vi "macro_DrumSeq_Pulse_Mux.vi"   [LabVIEW 2019, in "Trajectory_Library.lvlib"]
uses:
  VI/BoolCmd_Recv_Internal.vi
  VI/DigSeqLogic_Edge_On.vi
  VI/BoolCmd_ObtainQueue.vi
  Trajectory_Library.lvlib
types:
  T1 = typedef "Trajectory_Library.lvlib/DrumSequence_Step_Enum.ctl" = enum16{"Do Nothing", "Step 1", "Step 2", "Step 3", "Step 4", "Step 5", "Step 6", "Step 7", "Step 8", "Step 9", "Step 10", "Step 11", "Step 12", "Step 13", "Step 14", "Step 15", "Step 16", "Step 17", "Step 18", "Step 19", "Step 20", "Step 21", "Step 22", "Step 23", "Step 24", "Step 25", "Step 26", "Step 27", "Step 28", "Step 29", "Step 30", "Step 31", "Step 32", "Cancel", "Initialize", "Error"}
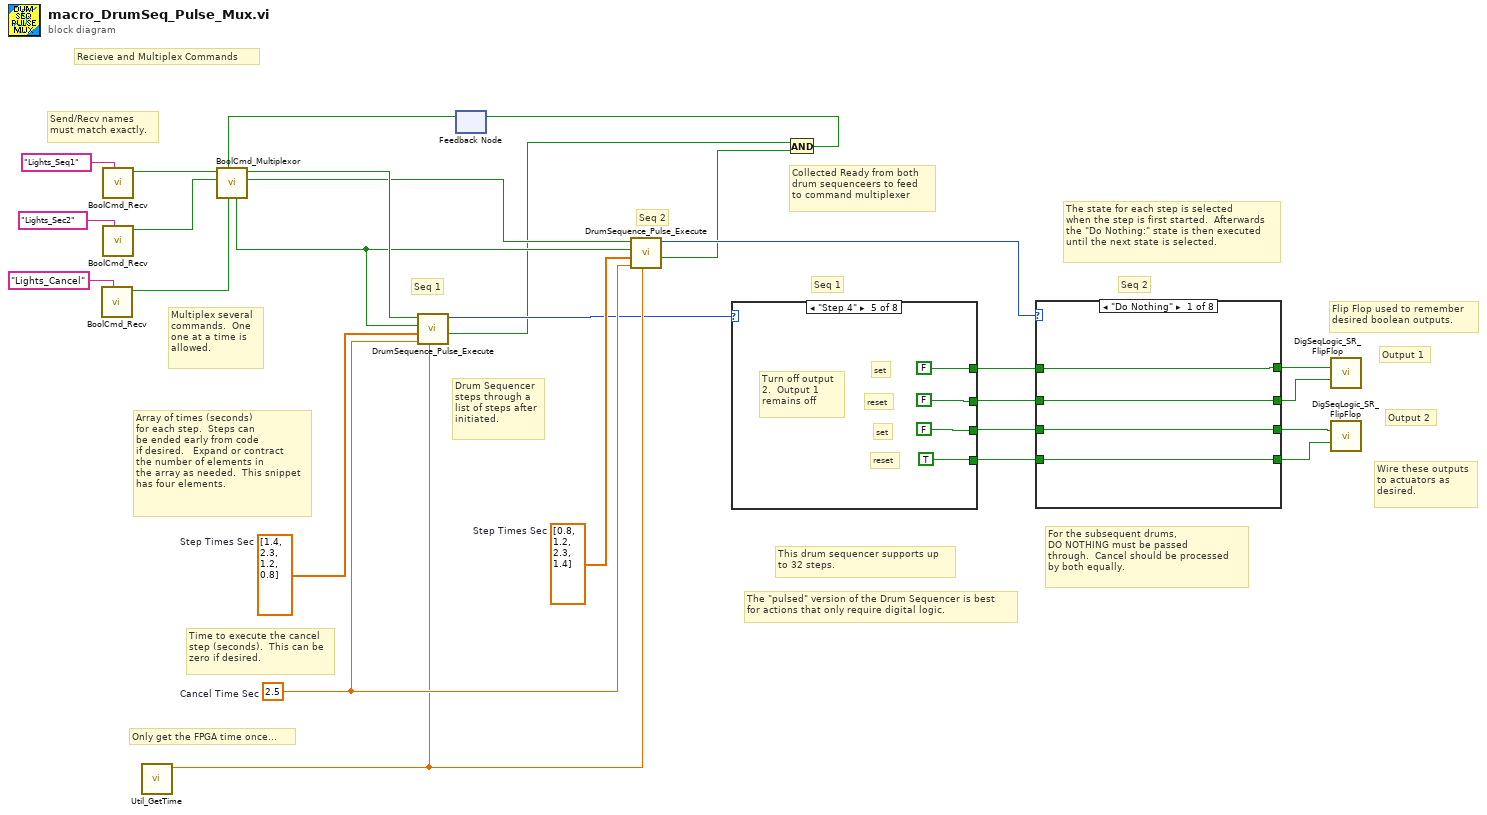
[diagram p0: block diagram]
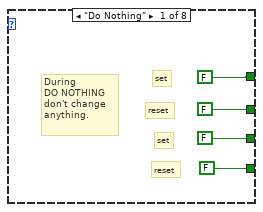
[diagram p2: hidden frame]
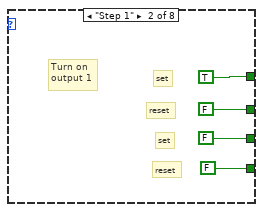
[diagram p3: hidden frame]
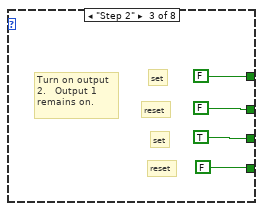
[diagram p4: hidden frame]
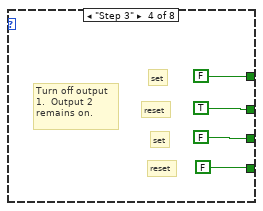
[diagram p5: hidden frame]
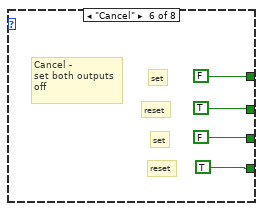
[diagram p6: hidden frame]
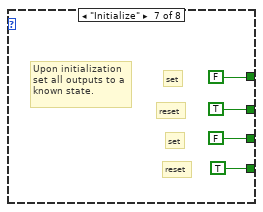
[diagram p7: hidden frame]
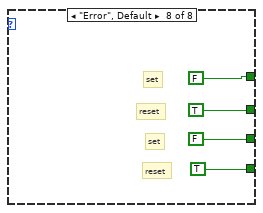
[diagram p8: hidden frame]
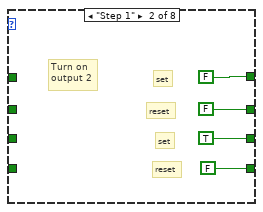
[diagram p9: hidden frame]
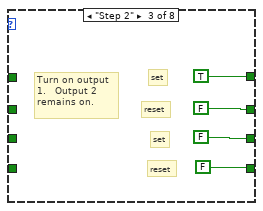
[diagram p10: hidden frame]
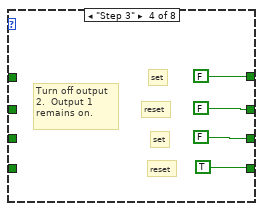
[diagram p11: hidden frame]
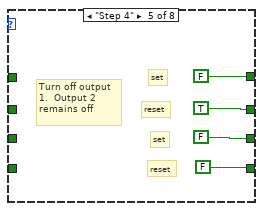
[diagram p12: hidden frame]
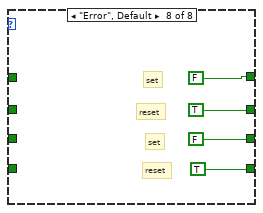
[diagram p15: hidden frame]
diagram:
  w10 = dbl[] [0.8, 1.2, 2.3, 1.4]  # Step Times Sec
  w9 = 2.5  # Cancel Time Sec
  w19 = dbl[] [1.4, 2.3, 1.2, 0.8]  # Step Times Sec
  # "Seq 2"
  # "Seq 1"
  # "Only get the FPGA time once..."
  # "For the subsequent drums, \nDO NOTHING must be passed\nthrough.  Cancel should be processed\nby both equally."
  # "Seq 2"
  # "Seq 1"
  # "This drum sequencer supports up\nto 32 steps."
  # "Wire these outputs\nto actuators as\ndesired."
  # "Output 2"
  # "Output 1"
  # "Flip Flop used to remember\ndesired boolean outputs."
  # "The \"pulsed\" version of the Drum Sequencer is best\nfor actions that only require digital logic."
  # "The state for each step is selected\nwhen the step is first started.  Afterwards\nthe \"Do Nothing:\" state is then executed\nuntil the next state is selected."
  # "Drum Sequencer\nsteps through a \nlist of steps after\ninitiated."
  # "Time to execute the cancel\nstep (seconds).  This can be\nzero if desired."
  # "Array of times (seconds)\nfor each step.  Steps can\nbe ended early from code\nif desired.   Expand or contract\nthe number of elements in\nthe array as needed.  This snippet\nhas four elements."
  # "Collected Ready from both\ndrum sequenceers to feed\nto command multiplexer"
  # "Multiplex several\ncommands.  One\none at a time is \nallowed."
  # "Send/Recv names\nmust match exactly."
  # "Recieve and Multiplex Commands"
  n1 = call "BoolCmd_Recv.vi"("Command Name"="Lights_Cancel") -> ("New Request"=w22:bool)  [unwired: 9 in, 1 out]
  n2 = call "BoolCmd_Recv.vi"("Command Name"="Lights_Seq1") -> ("New Request"=w24:bool)  [unwired: 9 in, 1 out]
  n3 = call "BoolCmd_Recv.vi"("Command Name"="Lights_Sec2") -> ("New Request"=w23:bool)  [unwired: 9 in, 1 out]
  n4 = call "Util_GetTime.vi"() -> ("FPGA_Time_Seconds"=w8:dbl)  [unwired: 9 in, 2 out]
  n5 = feedback #1() -> (w20:bool)  [unwired: 1 in]
  n6 = call "BoolCmd_Multiplexor.vi"("Command Cancel"=w22, "Ready"=w20, "Command 2"=w23, "Command 1"=w24) -> ("Do Command 2"=w4:bool, "Do Command 1"=w5:bool, "Do Cancel"=w3:bool)  [unwired: 3 in, 2 out]
  n7 = call "DrumSequence_Pulse_Execute.vi"("Pass_Through_Time"=w8, "Cancel Time Sec"=w9, "Step Times Sec"=w19, "Cancel"=w3, "Initiate"=w5) -> ("Ready"=w1:bool, "Step Number State"=w6:T1)  [unwired: 3 in, 2 out]
  n8 = call "DrumSequence_Pulse_Execute.vi"("Pass_Through_Time"=w8, "Cancel Time Sec"=w9, "Step Times Sec"=w10, "Cancel"=w3, "Initiate"=w4) -> ("Ready"=w2:bool, "Step Number State"=w7:T1)  [unwired: 3 in, 2 out]
  n9 = case shown="\"Step 4\"" w6 {
    tunnel: [FALSE TRUE FALSE FALSE FALSE FALSE FALSE FALSE] -> w14
    tunnel: [FALSE FALSE FALSE TRUE FALSE TRUE TRUE TRUE] -> w13
    tunnel: [FALSE FALSE TRUE FALSE FALSE FALSE FALSE FALSE] -> w12
    tunnel: [FALSE FALSE FALSE FALSE TRUE TRUE TRUE TRUE] -> w11
    frame "Do Nothing" {
      # "During \nDO NOTHING\ndon't change\nanything."
      # "reset"
      # "set"
      # "reset"
      # "set"
    }
    frame "Step 1" {
      # "Turn on \noutput 1"
      # "reset"
      # "set"
      # "reset"
      # "set"
    }
    frame "Step 2" {
      # "Turn on output\n2.   Output 1\nremains on."
      # "reset"
      # "set"
      # "reset"
      # "set"
    }
    frame "Step 3" {
      # "Turn off output\n1.  Output 2\nremains on."
      # "reset"
      # "set"
      # "reset"
      # "set"
    }
    frame "Step 4" {
      # "Turn off output\n2.  Output 1\nremains off"
      # "reset"
      # "set"
      # "reset"
      # "set"
    }
    frame "Cancel" {
      # "Cancel - \nset both outputs\noff"
      # "reset"
      # "set"
      # "reset"
      # "set"
    }
    frame "Initialize" {
      # "reset"
      # "set"
      # "reset"
      # "set"
      # "Upon initialization\nset all outputs to a\nknown state."
    }
    frame "Error", Default {
      # "reset"
      # "set"
      # "reset"
      # "set"
    }
  }
  n10 = And(x=w1, y=w2) -> (x .and. y?=w21:bool)
  n11 = feedback-in #1(w21) -> ()
  n12 = case shown="\"Do Nothing\"" w7 {
    tunnel: [w63 FALSE TRUE FALSE FALSE w83 w87 FALSE] -> w18
    tunnel: [w62 FALSE FALSE FALSE TRUE w82 w86 TRUE] -> w17
    tunnel: [w61 TRUE FALSE FALSE FALSE w81 w85 FALSE] -> w16
    tunnel: [w60 FALSE FALSE TRUE FALSE w80 w84 TRUE] -> w15
    tunnel: w14 -> [w63 _ _ _ _ w83 w87 _]
    tunnel: w13 -> [w62 _ _ _ _ w82 w86 _]
    tunnel: w12 -> [w61 _ _ _ _ w81 w85 _]
    tunnel: w11 -> [w60 _ _ _ _ w80 w84 _]
    frame "Do Nothing" {
    }
    frame "Step 1" {
      # "Turn on \noutput 2"
      # "reset"
      # "set"
      # "reset"
      # "set"
    }
    frame "Step 2" {
      # "Turn on output\n1.   Output 2\nremains on."
      # "reset"
      # "set"
      # "reset"
      # "set"
    }
    frame "Step 3" {
      # "Turn off output\n2.  Output 1\nremains on."
      # "reset"
      # "set"
      # "reset"
      # "set"
    }
    frame "Step 4" {
      # "Turn off output\n1.  Output 2\nremains off"
      # "reset"
      # "set"
      # "reset"
      # "set"
    }
    frame "Cancel" {
    }
    frame "Initialize" {
    }
    frame "Error", Default {
      # "reset"
      # "set"
      # "reset"
      # "set"
    }
  }
  n13 = call "DigSeqLogic_SR_FlipFlop.vi"("Set"=w18, "Reset"=w17) -> ()  [unwired: 12 in, 2 out]
  n14 = call "DigSeqLogic_SR_FlipFlop.vi"("Set"=w16, "Reset"=w15) -> ()  [unwired: 12 in, 2 out]
